vi "PH_Beamline.Calc MA State.vi"(0 "i ref in":refnum<vi>, 2 "PA Exit closed or shining into LL":bool, 5 "error in (no error)":errorcluster) -> (14 "i ref out":refnum<vi>, 19 "error out":errorcluster)   [LabVIEW 2014, in "PH_Beamline.lvlib"]
doc: "THIS VI calculates the MainAmp state of the Beamline"
uses:
  PH_Beamline.lvlib
  PH_StatusHandler/PH_StatusHandler.Status.ctl
  PH_Beamline.6P 4 Pos Selector Instances.ctl
  PH_4_Pos_Selector/PH_4_Pos_Selector.Position Selector.ctl
  PH_Common/PH_Common.lvlib
  PH_StatusHandler/PH_StatusHandler.lvlib
  PH_BL-Master/PH_BL-Master.lvlib
  PH_4_Pos_Selector/PH_4_Pos_Selector.lvlib
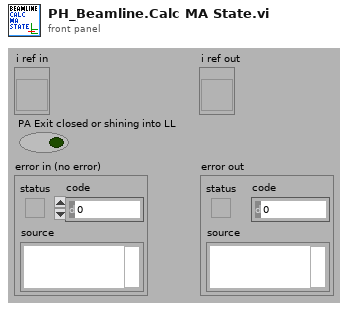
[diagram p1: front panel]
types:
  T1 = typedef "PH_Beamline.lvlib/PH_Beamline.i attribute.ctl" = cluster{"GUI Refs":cluster{"PA ok":refnum<vi>, "MA ok":refnum<vi>, "fs FE ok":refnum<vi>, "ns FE ok":refnum<vi>, "PA ED ok":refnum<vi>, "MAS ok":refnum<vi>, "Booster ok":refnum<vi>, "Mirrortower ok":refnum<vi>, "In.-Box ok":refnum<vi>, "Compressor ok":refnum<vi>, "Experiment LB ok":refnum<vi>, "Experiment LL ok":refnum<vi>, "PHELIX_Beckhoff_Watchdog":refnum<vi>, "Shutters closed":refnum<vi>, "uOPA ok":refnum<vi>, "Vacuum no shotcond Comp LB":refnum<vi>}, "Refs BL MA":refnum<vi>[], "Refs BL MA-IB":refnum<vi>[], "Refs BL fs":refnum<vi>[], "Refs BL PA ED":refnum<vi>[], "Refs BL MAS":refnum<vi>[], "Refs BL Boo":refnum<vi>[], "Refs BL ns":refnum<vi>[], "Refs BL Mirrortower":refnum<vi>[], "Refs BL Compressor":refnum<vi>[], "Refs BL Exp LB":refnum<vi>[], "Radiation Safety":cluster{"Exp Laserbay":cluster{"Ref Op Mode":refnum<vi>, "Ref Laserbay evacuated":refnum<vi>, "Tagname LB evacuated":string, "Shot Mode":T2, "Laserbay evacuated?":i32, "Tagname HV room locked":string, "HV room locked?":i32, "Ref HV room locked":refnum<vi>, "Tagname bridged?":string, "Ref Bridge":refnum<vi>, "I<1E18W/cm²":bool}, "Exp Laserlab":cluster{"Ref Op Mode":refnum<vi>, "Ref Laserlab evacuated":refnum<vi>, "Tagname LL evacuated":string, "Shot Mode":T2, "Laserlab evacuated?":i32, "Tagname bridged?":string, "Ref Bridge":refnum<vi>, "I<1E18W/cm²":bool}}, "Refs BL LL":refnum<vi>[], "PP Igni Heating GUI Refs":refnum<vi>[], "PP Igni Heating Tagnames ":string[], "Refs BL PA":cluster{"undelayed Line before Shutter":refnum<vi>[], "undelayed Line after Shutter":refnum<vi>[], "before Bypass":refnum<vi>[], "delayed Line before Shutter":refnum<vi>[], "delayed Line after Shutter":refnum<vi>[], "before Shutter Input":refnum<vi>[], "after Shutter Input":refnum<vi>[], "Bypass":refnum<vi>[], "before Shutter Exit":refnum<vi>[], "after Shutter Exit":refnum<vi>[], "to MA":refnum<vi>[], "to Lab":refnum<vi>[]}, "BL":cluster{"YLF_BL_Status":i32, "fs_BL_Status":i32, "fs_YLF_BL_Status":i32, "ns_BL_Status":i32, "PA_Input_BL_Status":i32, "PA_UnDelay_BL_Status":i32, "PA_Delay_BL_Status":i32, "PA_BL_Status":i32, "PA_Bypass_BL_Status":i32, "PA_Exit_BL_Status":i32, "PA_LL_BL_Status":i32, "LL_BL_Status":i32, "PA_MA_BL_Status":i32, "MA_Exit_BL_Status":i32, "MA_Z6_BL_Status":i32, "Z6_BL_Status":i32, "MA_LB_BL_Status":i32, "LB_TB2_BL_Status":i32, "PA_before_Bypass_BL_Status":i32, "LB_TB3_BL_Status":i32}, "State Subsystems":cluster{"PA":bool, "MA":bool, "ns FE":bool, "fs FE":bool, "PA ED":bool, "In.-Box":bool, "MAS":bool, "Booster":bool, "Mirrortower":bool, "Compressor":bool, "Experiment LB":bool, "Experiment LL":bool, "uOPA":bool}, "Status Subscriber Information":T3, "Refs BL uOPA":refnum<vi>[], "PA_Input_2_Beam_6PWpGUI not linked?":bool, "PA_Input_Delay_6PGUI not linked?":bool, "Settings":T6}
  T2 = typedef "PH_Beamline.lvlib/PH_Beamline.Operation Mode.ctl" = i32
  T3 = typedef "PH_Beamline.lvlib/PH_Beamline.Status Subscriber Information.ctl" = cluster{"fs Swich YLF":T4, "fs Exit Shutter":T4, "ns Exit Shutter":T4, "PA Input Shutter":T4, "PA PC WP":T4, "PA PC WP 2":T4, "PA Bypass In":T4, "PA Bypass Out":T4, "PA CH 1":T4, "PA delayed":T4, "PA non delayed":T4, "PA Exit Shutter":T4, "PA Switch Lab":T4, "PA Bridge CH Input MA":T4, "MA Diffusor IB":T4, "MA IB Ready":T4, "MA CH 1":T4, "MA CH 2":T4, "MA CH 3":T4, "MA CH 4":T4, "MA Shutter Align Cam":T4, "MA Position MM5":T4, "Calorimeter Switch":T4, "BL Z6 CH 9":T4, "BL Z6 Beamdump":T4, "BL Z6 Shutter":T4, "COS Sensitivity Switch":T4, "Exp LB Shutter":T4, "Exp LB TB 2":T4, "Exp LB TB 3":T4, "PA LL Input CH":T4, "PA LL Output CH":T4, "LL Comp Input Shutter":T4, "LL Comp Output Shutter":T4, "LL Comp FF Shutter":T4, "Exp LL Shutter":T4, "MA IM In IB":T4, "MA IM Out IB":T4, "MA DB In IB":T4, "MA DB Out IB":T4, "Exp LB Shutter Interlock":T4, "Exp LL Shutter Interlock":T4, "MM1 Force Sensor":T4}
  T4 = typedef "PH_BL-Master.lvlib/PH_BL-Master.Status Subscriber Information.ctl" = cluster{"Index of element":i32, "Attributeset":T5}
  T5 = typedef "PH_BL-Master.lvlib/PH_BL-Master.Attribute Set.ctl" = enum16{"Boolean Status Service Subscriber", "Picture Status Service Subscriber"}
  T6 = typedef "PH_Beamline_Chief.lvlib/PH_Beamline_Chief.Settings.ctl" = cluster{"PA Doublepass Mode":bool, "Compressor Vaccuum LB not relevant":bool, "Windowshutter TB2 not relevant":bool, "Windowshutter TB3 not relevant":bool}
  T7 = typedef "PH_Beamline.lvlib/PH_Beamline.6P 4 Pos Selector Instances.ctl" = string
  T8 = enum16{"All, Default", "PreAmp", "MainAmp", "Compressor", "Experiment", "Z6 Telescope"}
  T9 = typedef "PH_4_Pos_Selector.lvlib/PH_4_Pos_Selector.Position Selector.ctl" = u16
  T10 = typedef "PH_StatusHandler.lvlib/PH_StatusHandler.Status.ctl" = i16
  T11 = typedef "PH_BL-Master.lvlib/PH_BL-Master.i attribute.ctl" = cluster{"Remote controlled":bool, "Boolean Condition Service Subscriber":refnum<vi>[], "Picture Condition Service Subscriber":refnum<vi>[], "R2S":cluster{"GUI Ref":refnum<vi>, "State":bool}, "Vacua":cluster{"GUI Ref":refnum<vi>, "Limit":dbl, "Curr Value":dbl, "in range":bool}[], "O2 Inspection":cluster{"GUI Ref":refnum<vi>, "Concentration":dbl, "State":T10}[], "Boolean Status Service Subscriber":cluster{"GUI Ref":refnum<vi>, "Status":T10, "no Link?":bool, "Status Subscriber Class":T12}[], "Picture Status Service Subscriber":cluster{"GUI Ref":refnum<vi>, "Status":T10, "no Link?":bool, "Status Subscriber Class":T12}[], "6P 4Q Service Subscriber":cluster{"GUI Ref":refnum<vi>, "Selector":T9, "no Link?":bool}[], "Index of latest 6P 4Q changing Instance":i32, "Index of latest Picture Status changing Instance":i32, "Index of latest Boolean Status changing Instance":i32, "Vision ID on same Node":string, "Start Phase over?":bool, "GUI Ref Delete":refnum<vi>}
  T12 = typedef "PH_BL-Master.lvlib/PH_BL-Master.Status Subscriber Class.ctl" = enum16{"unknown", "Switch", "BB", "6P Switch", "Switch GUI", "Switch and 6P State", "Force Sensor"}
  T13 = cluster{"GUI Ref":refnum<vi>, "Concentration":dbl, "State":T10}[]
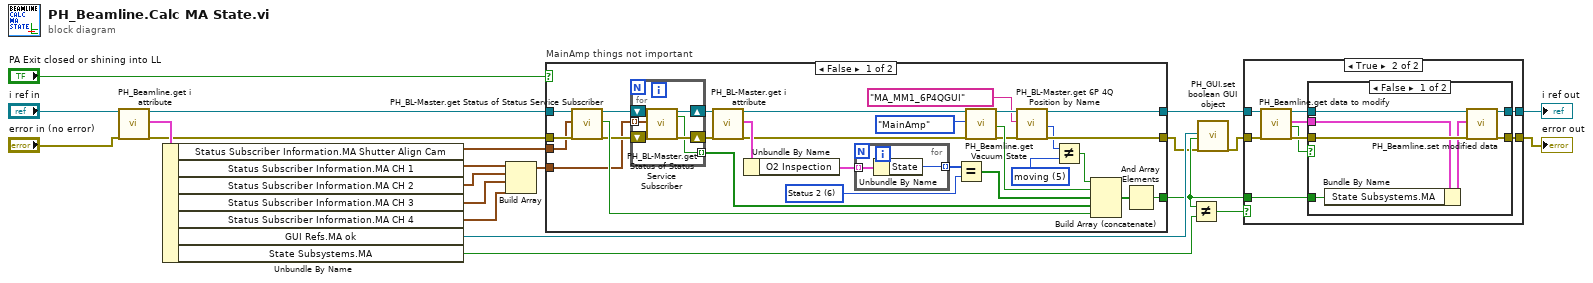
[diagram p0: block diagram]
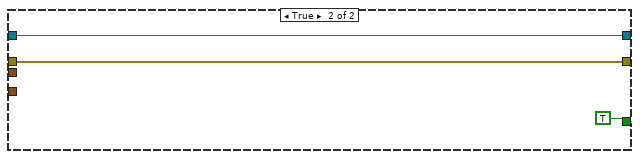
[diagram p4: hidden frame]
diagram:
  n1 = call "PH_Beamline.get i attribute.vi"("i ref in"="i ref in", "error in (no error)"="error in (no error)") -> ("i ref out"=w1:refnum<vi>, "i attribute"=w21:T1, "error out"=w2:errorcluster)  [unwired: 15 in]
  n2 = Unbundle By Name(w21) -> ("Status Subscriber Information.MA Shutter Align Cam"=w9:T4, "Status Subscriber Information.MA CH 1"=w8:T4, "Status Subscriber Information.MA CH 2"=w7:T4, "Status Subscriber Information.MA CH 3"=w6:T4, "Status Subscriber Information.MA CH 4"=w5:T4, "GUI Refs.MA ok"=w20:refnum<vi>, "State Subsystems.MA"=w15:bool)
  n3 = Build Array(w8, w7, w6, w5) -> (w4:T4[])
  n4 = case "MainAmp things not important" shown="False" "PA Exit closed or shining into LL" {
    tunnel: w1 -> [w40 w61]
    tunnel: [w26 w61] -> w11
    tunnel: w2 -> [w39 w60]
    tunnel: [w28 w60] -> w10
    tunnel: [w48 TRUE] -> w14
    tunnel: w9 -> [w31 _]
    tunnel: w4 -> [w30 _]
    frame False {
      w24 = T9 5 items=["unknown", "Position I", "Position II", "Position III", "Position IV", "moving"] ("y")
      w45 = T10 6 items=["no info", "off/false/out", "on/true/in", "Failure", "Alarm", "Status 1", "Status 2", "Status 3"] ("State")
      n5 = call "PH_BL-Master.get Status of Status Service Subscriber.vi"("i ref in"=w40, "Wanted Status Subscriber Information"=w31, "error in (no error)"=w39) -> ("i ref out"=w37:refnum<vi>, "on/true/in?"=w43:bool, "error out"=w36:errorcluster)  [unwired: 11 in, 3 out]
      n6 = for {
        tunnel: [w53] -> w49 mode=indexing
        shift-right: [w57] -> w35
        shift-left: w37 -> [w58]
        shift-right: [w55] -> w33
        shift-left: w36 -> [w56]
        tunnel: w30 -> [w54] mode=indexing
        n7 = call "PH_BL-Master.get Status of Status Service Subscriber.vi"("i ref in"=w58, "Wanted Status Subscriber Information"=w54, "error in (no error)"=w56) -> ("i ref out"=w57:refnum<vi>, "off/false/out?"=w53:bool, "error out"=w55:errorcluster)  [unwired: 11 in, 3 out]
      }
      n8 = call "PH_BL-Master.get i attribute.vi"("i ref in"=w35, "error in (no error)"=w33) -> ("i ref out"=w34:refnum<vi>, "i attribute"=w42:T11, "error out"=w32:errorcluster)  [unwired: 15 in]
      n9 = Unbundle By Name(w42) -> ("O2 Inspection"=w47:T13)
      n10 = for {
        tunnel: w47 -> [w52] mode=indexing
        tunnel: [w51] -> w46 mode=indexing
        n11 = Unbundle By Name(w52) -> ("State"=w51:T10)
      }
      n12 = Equal?(x=w46, y=w45) -> (x = y?=w41:bool[])
      n13 = call "PH_Beamline.get Vacuum State.vi"("i ref in"=w34, "Subsystem"=T8."MainAmp", "error in (no error)"=w32) -> ("i ref out"=w27:refnum<vi>, "vacua in range"=w38:bool, "error out"=w29:errorcluster)  [unwired: 14 in]
      n14 = call "PH_BL-Master.get 6P 4Q Position by Name.vi"("i ref in"=w27, "6P 4Q Instance"=T7 "MA_MM1_6P4QGUI", "error in (no error)"=w29) -> ("i ref out"=w26:refnum<vi>, "Position"=w23:T9, "error out"=w28:errorcluster)  [unwired: 10 in, 4 out]
      n15 = Not Equal?(x=w23, y=w24) -> (x != y?=w22:bool)
      n16 = Build Array (concatenate)(w22, w38, w41, w49, w43) -> (w50:bool[])
      n17 = And Array Elements(Boolean array=w50) -> (logical AND=w48:bool)
    }
    frame True {
    }
  }
  n18 = Not Equal?(x=w14, y=w15) -> (x != y?=w19:bool)
  n19 = call "PH_GUI.set boolean GUI object.vi"("Boolean Knob GUI Ref"=w20, "Value"=w14, "error in (no error)"=w10) -> ("error out"=w18:errorcluster)  [unwired: 16 in]
  n20 = case shown="True" w19 {
    tunnel: w11 -> [w63 w68]
    tunnel: [w63 w67] -> w16
    tunnel: w18 -> [w62 w66]
    tunnel: [w62 w65] -> w17
    tunnel: w14 -> [_ w64]
    frame False {
    }
    frame True {
      n21 = call "PH_Beamline.get data to modify.vi"("i ref in"=w68, "error in (no error)"=w66) -> ("i ref out"=w71:refnum<vi>, "i attribute"=w69:T1, "timed out"=w70:bool, "error out"=w72:errorcluster)  [unwired: 14 in]
      n22 = case shown="False" w70 {
        tunnel: w72 -> [w79 w80]
        tunnel: w71 -> [w78 w81]
        tunnel: [w77 w80] -> w65
        tunnel: [w76 w81] -> w67
        tunnel: w69 -> [w75 _]
        tunnel: w64 -> [w73 _]
        frame False {
          n23 = Bundle By Name(cluster=w75, "State Subsystems.MA"=w73) -> (w74:T1)
          n24 = call "PH_Beamline.set modified data.vi"("i ref in"=w78, "i attribute"=w74, "error in (no error)"=w79) -> ("i ref out"=w76:refnum<vi>, "error out"=w77:errorcluster)  [unwired: 15 in]
        }
        frame True {
        }
      }
    }
  }
  "i ref out" <- w16
  "error out" <- w17
